vi "read_auto_file.vi"(0 "File Name With Extension":string) -> (1 "File Contents":string, 2 "error out":errorcluster)   [LabVIEW 2015]
uses:
  Auto_Conf.vi
  <vilib>/Rock Robotics/Network Tables/SD Write String.vi
panel:
  out "lowercase file extension":string
  out "file or folder exists?":bool
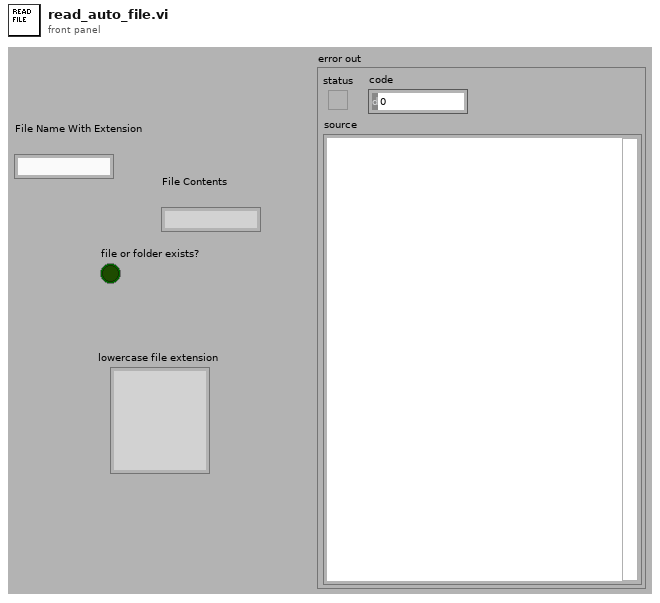
[diagram p1: front panel]
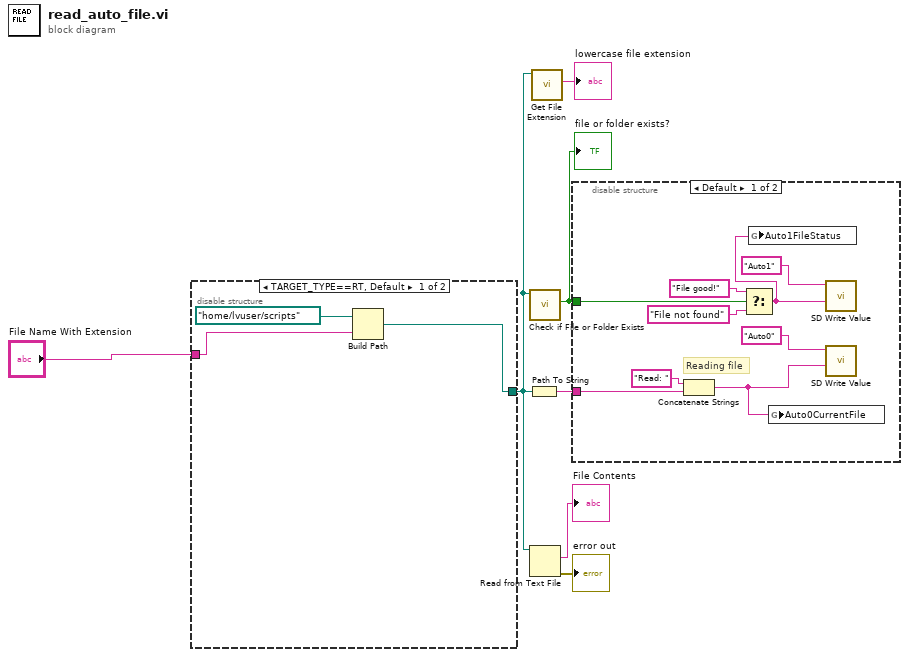
[diagram p0: block diagram]
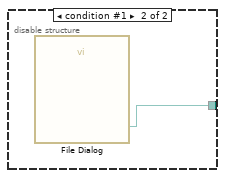
[diagram p3: hidden frame]
diagram:
  n1 = disable-structure shown="TARGET_TYPE==RT, Default" {
    disable-tunnel: "File Name With Extension" -> [w10 _]
    disable-tunnel: [w8 w11] -> w1
    frame condition #0 (active) {
      n2 = Build Path(base path=path "/home/lvuser/scripts", name or relative path=w10) -> (appended path=w8:path)
    }
    frame condition #1 {
      n3 = call "File Dialog"() -> ("selected path"=w11:path)  [unwired: 7 in, 8 out]
    }
  }
  n4 = Path To String(path=w1) -> (string=w3:string)
  n5 = call <vilib>:"Check if File or Folder Exists.vi"("path"=w1) -> ("file or folder exists?"=w4:bool)  [unwired: 1 in, 9 out]
  "file or folder exists?" <- w4
  n6 = Read from Text File(file (use dialog)=w1) -> (text=→"File Contents":string, error out=→"error out":errorcluster)  [unwired: 1 in, 4 out]
  n7 = call <vilib>:"Get File Extension.vi"("file"=w1) -> ("lowercase file extension"=→"lowercase file extension":string)  [unwired: 1 in, 9 out]
  n8 = disable-structure shown="Default" {
    disable-tunnel: w4 -> [w20 _]
    disable-tunnel: w3 -> [w16 _]
    frame condition #0 (active) {
      # "Reading file"
      n9 = Concatenate Strings("Read: " ("string"), w16) -> (w13:string)
      n10 = Select(t="File good!", s=w20, f="File not found") -> (s? t:f=w12:string)
      n11 = global write "Auto_Conf.vi" "Auto1FileStatus"(w12) -> ()
      n12 = global write "Auto_Conf.vi" "Auto0CurrentFile"(w13) -> ()
      n13 = call-poly <vilib>:"SD Write Value.vi"("String"=w12, "Name"="Auto1") -> ()  [unwired: 8 in, 2 out]
      n14 = call-poly <vilib>:"SD Write Value.vi"("String"=w13, "Name"="Auto0") -> ()  [unwired: 8 in, 2 out]
    }
    frame condition #1 {
    }
  }
